vi "GyroActions.vi"(9 "RobotFront":bool, 10 "Update?":bool, 11 "Zero":bool) -> (0 "Yaw":dbl, 3 "YRPHfH":T1)   [LabVIEW 2018]
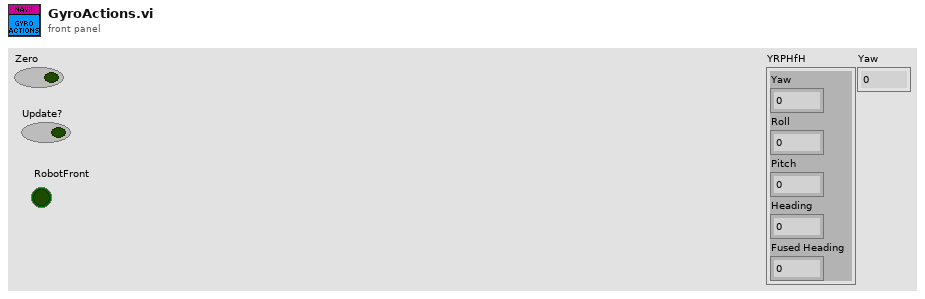
[diagram p1: front panel]
types:
  T1 = cluster{"Yaw":dbl, "Roll":dbl, "Pitch":dbl, "Heading":dbl, "Fused Heading":dbl}
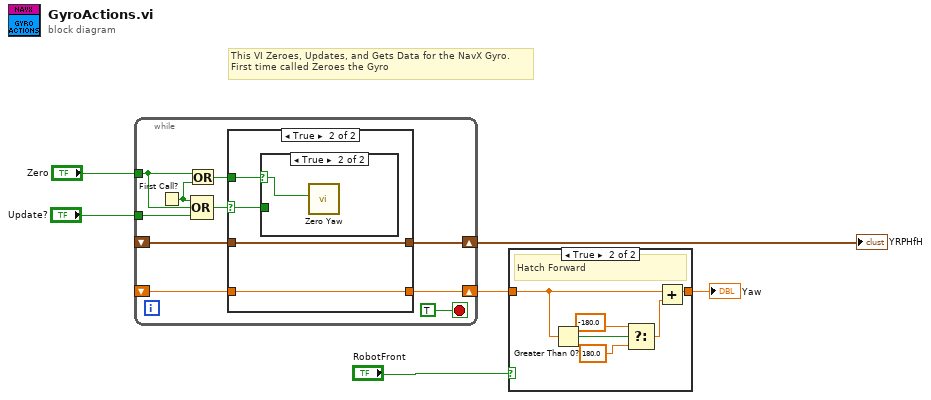
[diagram p0: block diagram]
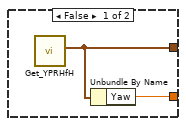
[diagram p3: hidden frame]
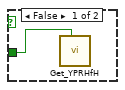
[diagram p4: hidden frame]
diagram:
  # "This VI Zeroes, Updates, and Gets Data for the NavX Gyro.\nFirst time called Zeroes the Gyro"
  n1 = while {
    tunnel: "Zero" -> [w13]
    tunnel: "Update?" -> [w12]
    shift-right: [w10] -> w4
    shift-left: _ -> [w8]
    shift-right: [w9] -> w2
    shift-left: _ -> [w7]
    stop <- TRUE stop-if-true
    n2 = First Call?() -> (First Call?: T/F=w14:bool)
    n3 = Or(x=w13, y=w14) -> (x .or. y?=w15:bool)
    n4 = Compound Arithmetic op=OR(w14, w13, w12) -> (w11:bool)
    n5 = case shown="True" w11 {
      selector: w11 -> [_ w21]
      tunnel: w15 -> [_ w22]
      tunnel: [w18 w20] -> w10
      tunnel: [w17 w19] -> w9
      tunnel: w8 -> [_ w20]
      tunnel: w7 -> [_ w19]
      frame False {
        n6 = call <vilib>:"Get_YPRHfH.vi"() -> ("YRPHfH"=w18:T1)  [unwired: 11 in]
        n7 = Unbundle By Name(w18) -> ("Yaw"=w17:dbl)
      }
      frame True {
        n8 = case shown="True" w22 {
          selector: w22 -> [_ w24]
          tunnel: w21 -> [w23 _]
          frame False {
            n9 = call <vilib>:"Get_YPRHfH.vi"("Update"=w23) -> ()  [unwired: 10 in, 1 out]
          }
          frame True {
            n10 = call <vilib>:"Zero Yaw.vi"("Zero"=w24) -> ()  [unwired: 11 in]
          }
        }
      }
    }
  }
  "YRPHfH" <- w4
  n11 = case shown="True" "RobotFront" {
    tunnel: [w25 w31] -> w3
    tunnel: w2 -> [w25 w30]
    frame False {
      # "Torros Forward"
    }
    frame True {
      # "Hatch Forward"
      n12 = Greater Than 0?(x=w30) -> (x > 0?=w29:bool)
      n13 = Select(t=-180.0, s=w29, f=180.0 ("y")) -> (s? t:f=w26:dbl)
      n14 = Add(x=w30, y=w26) -> (x+y=w31:dbl)
    }
  }
  "Yaw" <- w3
